vi "Example Graph - Acceleration Callback.vi"(4 "Acceleration":refnum<user-event>, 5 "Event Data":T1, 6 "Control Ref":refnum<k24>, 7 "Event Common Data":T2) -> ()   [LabVIEW 2010]
uses:
  C:/tf/play/labview/Tinkerforge.dll
  Tinkerforge.dll
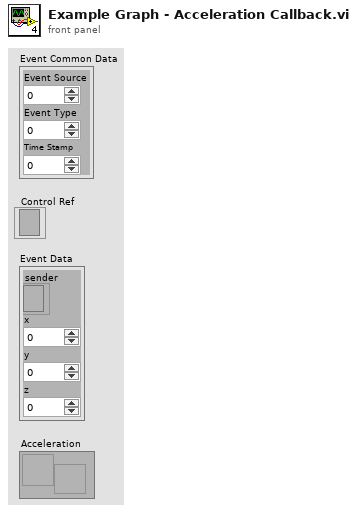
[diagram p1: front panel]
types:
  T1 = cluster{"sender":refnum<k24>, "x":i16, "y":i16, "z":i16}
  T2 = cluster{"Event Source":i32, "Event Type":u32, "Time Stamp":u32}
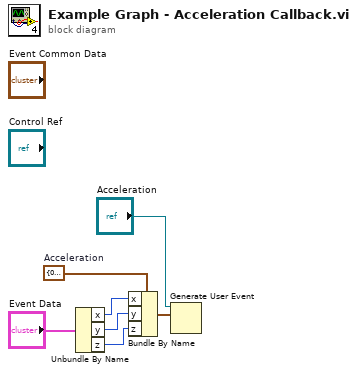
[diagram p0: block diagram]
diagram:
  w6 = cluster{"x":i16, "y":i16, "z":i16} {"x"=0, "y"=0, "z"=0}  # Acceleration
  n1 = Unbundle By Name("Event Data") -> ("x"=w5:i16, "y"=w4:i16, "z"=w3:i16)
  n2 = Bundle By Name(cluster=w6, "x"=w5, "y"=w4, "z"=w3) -> (w1:cluster{"x":i16, "y":i16, "z":i16})
  n3 = Generate User Event(user event="Acceleration", event data cluster=w1) -> ()  [unwired: 1 in, 2 out]
